vi "Main Tclk.vi"() -> ()   [LabVIEW 2018] (continued)
                        n6385 = invoke class="_EMApi" method="Execute"(reference=w1050, "lpszCommand"="CMD_FIB_TC_MH_REQ_START") -> ()  [unwired: 2 in, 4 out]
                      }
                      frame #2 {
                        n6386 = Wait (ms)(milliseconds to wait=u32 30000) -> ()  [unwired: 1 out]
                        n6387 = local write "Status message"("FIB reheat in progress..." ("Status message")) -> ()
                      }
                      frame #3 {
                        n6388 = while {
                          stop <- w1058 stop-if-true
                          n6389 = local read "Api"() -> (w1055:refnum<k7>)
                          n6390 = call "SmartSEM Remote API FIB gun state.vi"("ActiveX Container"=w1055) -> ("FIB Gun State"=w1057:string, "reference out"=w1053:refnum<k7>)  [unwired: 8 in, 1 out]
                          n6391 = Wait Until Next ms Multiple(millisecond multiple=u32 100) -> ()  [unwired: 1 out]
                          n6392 = case shown="\"FIB Emissin Failed\"" w1057 {
                            tunnel: [FALSE ("x") TRUE ("x") w1075] -> w1056
                            tunnel: w1053 -> [_ _ w1074]
                            frame "", Default {
                            }
                            frame "FIB Emissin Failed" {
                              n6393 = Get Date/Time In Seconds() -> (seconds since 1Jan1904=w1064:timestamp)
                              n6394 = Get Date/Time String(seconds (now)=w1064) -> (date string=w1065:string, time string=w1066:string)  [unwired: 2 in]
                              n6395 = Concatenate Strings(w1065, " " ("string"), w1066) -> (w1063:string)
                              n6396 = local read "Reheat Output"() -> (w1068:T21)
                              n6397 = Bundle By Name(cluster=w1068, "Reheat finish time"=w1063, "Reheat Success"=FALSE) -> (w1069:T21)
                              n6398 = local write "Reheat Output"(w1069) -> ()
                            }
                            frame "Regulating" {
                              n6399 = call "SmartSEM Remote API get string.vi"("lpszParam"="DP_FIB_PURGE_STATE", "ActiveX Container"=w1074) -> ("data"=w1072:string, "reference out"=w1071:refnum<k7>)  [unwired: 7 in, 1 out]
                              n6400 = case shown="\"Idle\"" w1072 {
                                tunnel: w1071 -> [_ w1078]
                                tunnel: [FALSE ("x") w1077] -> w1075
                                frame "", Default {
                                }
                                frame "Idle" {
                                n6401 = stacked-sequence {
                                tunnel: w1078 -> [w1081 _ w1086 _]
                                tunnel: [_ _ _ TRUE ("x")] -> w1077
                                frame #0 {
                                n6402 = local read "FIB HW Config"() -> (w1080:T23)
                                n6403 = Unbundle By Name(w1080) -> ("Beam blank"=w1079:tag)
                                n6404 = call "FIB beam blank.vi"("ActiveX Container"=w1081, "Beam blanked"=TRUE, "lines"=w1079) -> ()  [unwired: 2 in, 1 out]
                                }
                                frame #1 {
                                n6405 = Wait (ms)(milliseconds to wait=u32 60000) -> ()  [unwired: 1 out]
                                n6406 = local write "Status message"("Stablizing for 1 min ..." ("Status message")) -> ()
                                }
                                frame #2 {
                                n6407 = call "SmartSEM Remote API FIB VI slope.vi"("ActiveX Container"=w1086) -> ("V/I slope"=w1087:sgl)  [unwired: 8 in, 2 out]
                                n6408 = local write "Status message"("Measuring FIB V/I slope ..." ("Status message")) -> ()
                                n6409 = local write "FIB V/I slope"(w1087) -> ()
                                }
                                frame #3 {
                                }
                                }
                                }
                              }
                            }
                          }
                          n6410 = local read "Stop Reheat"() -> (w1054:bool)
                          n6411 = local read "Stop"() -> (w1060:bool)
                          n6412 = Compound Arithmetic op=OR(w1056, w1060, w1054) -> (w1058:bool)
                        }
                      }
                      frame #4 {
                        n6413 = while {
                          stop <- w1095 stop-if-true
                          n6414 = local read "Api"() -> (w1091:refnum<k7>)
                          n6415 = call "SmartSEM Remote API FIB gun state.vi"("ActiveX Container"=w1091) -> ("FIB Gun State"=w1094:string, "reference out"=w1089:refnum<k7>)  [unwired: 8 in, 1 out]
                          n6416 = Wait Until Next ms Multiple(millisecond multiple=u32 100) -> ()  [unwired: 1 out]
                          n6417 = case shown="\"Regulating\"" w1094 {
                            tunnel: [FALSE ("x") TRUE ("x") TRUE ("x") w1117] -> w1093
                            tunnel: w1089 -> [_ _ _ w1118]
                            frame "", Default {
                            }
                            frame "FIB Emissin Failed" {
                              n6418 = Get Date/Time In Seconds() -> (seconds since 1Jan1904=w1101:timestamp)
                              n6419 = Get Date/Time String(seconds (now)=w1101) -> (date string=w1102:string, time string=w1103:string)  [unwired: 2 in]
                              n6420 = Concatenate Strings(w1102, " " ("string"), w1103) -> (w1100:string)
                              n6421 = local read "Reheat Output"() -> (w1105:T21)
                              n6422 = Bundle By Name(cluster=w1105, "Reheat finish time"=w1100, "Reheat Success"=FALSE) -> (w1106:T21)
                              n6423 = local write "Reheat Output"(w1106) -> ()
                            }
                            frame "Standby" {
                              n6424 = Get Date/Time In Seconds() -> (seconds since 1Jan1904=w1110:timestamp)
                              n6425 = Get Date/Time String(seconds (now)=w1110) -> (date string=w1111:string, time string=w1112:string)  [unwired: 2 in]
                              n6426 = Concatenate Strings(w1111, " " ("string"), w1112) -> (w1109:string)
                              n6427 = local read "Reheat Output"() -> (w1114:T21)
                              n6428 = Bundle By Name(cluster=w1114, "Reheat finish time"=w1109, "Reheat Success"=FALSE) -> (w1115:T21)
                              n6429 = local write "Reheat Output"(w1115) -> ()
                            }
                            frame "Regulating" {
                              n6430 = stacked-sequence {
                                tunnel: w1118 -> [w1121 w1128]
                                tunnel: [_ w1129] -> w1117
                                frame #0 {
                                n6431 = Wait (ms)(milliseconds to wait=u32 2000) -> ()  [unwired: 1 out]
                                n6432 = call "SmartSEM Remote API set float.vi"("vValue"=sgl 1.0, "lpszParam"="DP_FIB_BLANKED", "ActiveX Container"=w1121) -> ("error out"=w1119:errorcluster, "reference out"=w1120:refnum<k7>)  [unwired: 7 in]
                                n6433 = call "SmartSEM Remote API get FIB HV data.vi"("error in"=w1119, "ActiveX Container"=w1120) -> ("Capella HV Data Output"=w1124:T17)  [unwired: 6 in, 3 out]
                                n6434 = local write "Capella HV Data Output"(w1124) -> ()
                                }
                                frame #1 {
                                n6435 = call "SmartSEM Remote API get string.vi"("lpszParam"="DP_FIB_PURGE_STATE", "ActiveX Container"=w1128) -> ("data"=w1126:string)  [unwired: 7 in, 2 out]
                                n6436 = case shown="\"Idle\"" w1126 {
                                tunnel: w1128 -> [_ w1132]
                                tunnel: [FALSE ("x") w1131] -> w1129
                                frame "", Default {
                                }
                                frame "Idle" {
                                n6437 = stacked-sequence {
                                tunnel: w1132 -> [_ w1143 _]
                                tunnel: [_ _ TRUE ("x")] -> w1131
                                frame #0 {
                                w1134 = TRUE ("Reheat Success")
                                n6438 = Get Date/Time In Seconds() -> (seconds since 1Jan1904=w1136:timestamp)
                                n6439 = local read "FIB V/I slope"() -> (w1133:sgl)
                                n6440 = Get Date/Time String(seconds (now)=w1136) -> (date string=w1137:string, time string=w1138:string)  [unwired: 2 in]
                                n6441 = Concatenate Strings(w1137, " " ("string"), w1138) -> (w1135:string)
                                n6442 = local read "Reheat Output"() -> (w1140:T21)
                                n6443 = Bundle By Name(cluster=w1140, "Reheat finish time"=w1135, "Reheat Success"=w1134, "V/I Slope"=w1133) -> (w1141:T21)
                                n6444 = local write "Start FIB HV DataLog"(w1134) -> ()
                                n6445 = local write "Reheat Output"(w1141) -> ()
                                }
                                frame #1 {
                                n6446 = call "SmartSEM Remote API FIB Gun Valve.vi"("FIB Gun Valve"=enum16{"Close", "Open"}."Open", "ActiveX Container"=w1143) -> ()  [unwired: 8 in, 2 out]
                                }
                                frame #2 {
                                n6447 = local read "Reheat Output"() -> (w1148:T21)
                                n6448 = local read "Capella HV Data Output"() -> (w1146:T17)
                                n6449 = Unbundle By Name(w1146) -> ("Emission Actual (uA)"=w1145:sgl, "Suppressor (V)"=w1144:sgl)
                                n6450 = Bundle By Name(cluster=w1148, "Initial emission (uA)"=w1145, "Initial suppressor (V)"=w1144) -> (w1147:T21)
                                n6451 = local write "Reheat Output"(w1147) -> ()
                                }
                                }
                                }
                                }
                                }
                              }
                            }
                          }
                          n6452 = local write "Status message"("Finishing FIB reheat ..." ("Status message")) -> ()
                          n6453 = local read "Stop Reheat"() -> (w1090:bool)
                          n6454 = local read "Stop"() -> (w1097:bool)
                          n6455 = Compound Arithmetic op=OR(w1093, w1097, w1090) -> (w1095:bool)
                        }
                      }
                      frame #5 {
                        n6456 = local read "Stop Reheat"() -> (w1150:bool)
                        n6457 = case shown="False" w1150 {
                          frame False {
                            n6458 = local read "Api"() -> (w1152:refnum<k7>)
                            n6459 = call "SmartSEM Remote API FIB HV offset removal.vi"("Max offset threshold (V)"=sgl 80.0, "ActiveX Container"=w1152) -> ("FIB HV matched"=w1151:bool)  [unwired: 8 in, 1 out]
                            n6460 = local write "FIB HV target matched"(w1151) -> ()
                          }
                          frame True {
                          }
                        }
                      }
                      frame #6 {
                        n6461 = local read "Stop Reheat"() -> (w1154:bool)
                        n6462 = case shown="False" w1154 {
                          tunnel: w1155 -> [w1157 w1162]
                          frame False {
                            n6463 = local read "Reheat Output"() -> (w1160:T21)
                            n6464 = local read "FIB Reheat Log Files"() -> (w1159:path)
                            n6465 = local read "Reheat time"() -> (w1158:timestamp)
                            n6466 = local read "Capella HV Data Output"() -> (w1156:T17)
                            n6467 = local write "Status message"("FIB reheat completed" ("Status message")) -> ()
                            n6468 = call "Write FIB reheat log.vi"("Capella HV Data Output"=w1156, "Reheat Output"=w1160, "Reheat time"=w1158, "Machine Type"=w1157, "Log file path"=w1159) -> ()  [unwired: 7 in]
                          }
                          frame True {
                            n6469 = local read "Reheat Output"() -> (w1165:T21)
                            n6470 = local read "FIB Reheat Log Files"() -> (w1164:path)
                            n6471 = local read "Reheat time"() -> (w1163:timestamp)
                            n6472 = local write "Status message"("FIB reheat stopped" ("Status message")) -> ()
                            n6473 = call "Write FIB reheat log.vi"("Reheat Output"=w1165, "Reheat time"=w1163, "Machine Type"=w1162, "Log file path"=w1164) -> ()  [unwired: 8 in]
                          }
                        }
                      }
                    }
                  }
                }
              }
              frame #2 {
                w1167 = u8 0 ("FIB emission below limit counts")
                w1170 = FALSE ("Start Reheat")
                n6474 = local write "Start Reheat"(w1170) -> ()
                n6475 = local write "Stop Reheat"(w1170) -> ()
                n6476 = local write "Turn FIB Gun on"(w1170) -> ()
                n6477 = property on="Request to stop reheat" class="Bool (strict)"("DisabledEnum"=T44."Disabled and Grayed Out" ("Disabled")) -> ()  [unwired: 2 in, 2 out]
                n6478 = local write "FIB emission limit warning armed"(TRUE ("FIB emission limit warning armed")) -> ()
                n6479 = local write "FIB emission below limit counts"(w1167) -> ()
                n6480 = local write "FIB suppressor below limit counts"(w1167) -> ()
                "Reheat completed" <- TRUE ("Reheat completed")
              }
            }
          }
        }
        n6481 = local read "Stop"() -> (w889:bool)
      }
      n6482 = while {
        stop <- w5736 stop-if-true
        n6483 = stacked-sequence {
          tunnel: [_ w5783] -> w5736
          frame #0 {
            n6484 = local read "Spot"() -> (w5739:bool)
            n6485 = shared-variable "My Computer\\Zeiss Library.lvlib\\Spot"(w5739) -> ()  [unwired: 1 in, 1 out]
            n6486 = local read "Machine Type"() -> (w5738:u8)
            n6487 = case shown="True" w5739 {
              tunnel: w5738 -> [_ w5741]
              frame False {
                n6488 = shared-variable ".\\Zeiss Library.lvlib\\FIB spot mode"(FALSE ("FIB spot mode")) -> ()  [unwired: 1 in, 1 out]
              }
              frame True {
                n6489 = stacked-sequence {
                  tunnel: w5741 -> [_ _ _ _ w5764 _ _]
                  frame #0 {
                    w5743 = 5.0 ("Cursor.Cursor Position:Cursor X")
                    w5742 = FALSE ("Unfreeze")
                    w5744 = TRUE ("Realtime Imaging stop")
                    n6490 = shared-variable "My Computer\\Zeiss Library.lvlib\\Realtime Imaging stop"(w5744) -> ()  [unwired: 1 in, 1 out]
                    n6491 = shared-variable ".\\Zeiss Library.lvlib\\FIB spot mode"(w5744) -> ()  [unwired: 1 in, 1 out]
                    n6492 = property on="FIB Imaging" class="Bool (strict)"("DisabledEnum"=T44."Disabled and Grayed Out" ("Disabled")) -> ()  [unwired: 2 in, 2 out]
                    n6493 = property on="FIB Image" class="IntGraph (strict)"() -> ("Width"=w5746:u32, "Height"=w5747:u32)  [unwired: 2 in, 2 out]
                    n6494 = expression code="x/2"(w5746) -> ()  [unwired: 1 out]
                    n6495 = expression code="x/2"(w5747) -> ()  [unwired: 1 out]
                    n6496 = local write "FIB Imaging"(w5742) -> ()
                    n6497 = local write "Unfreeze"(w5742) -> ()
                    n6498 = property on="FIB Image" class="IntGraph (strict)"("Cursor.Cursor X"=w5743, "Cursor.Cursor Y"=w5743) -> ()  [unwired: 2 in, 2 out]
                  }
                  frame #1 {
                    w5748 = -0.99 ("Spot X")
                    n6499 = Wait (ms)(milliseconds to wait=u32 500) -> ()  [unwired: 1 out]
                    n6500 = shared-variable ".\\Zeiss Library.lvlib\\Spot X"(w5748) -> ()  [unwired: 1 in, 1 out]
                    n6501 = shared-variable "My Computer\\Zeiss Library.lvlib\\Spot Z"(w5748) -> ()  [unwired: 1 in, 1 out]
                  }
                  frame #2 {
                    n6502 = local read "FIB HW Config"() -> (w5752:T23)
                    n6503 = local read "Api"() -> (w5750:refnum<k7>)
                    n6504 = local read "FIB Scan Parameters"() -> (w5751:T32)
                    n6505 = local read "FIB Options"() -> (w5756:T33)
                    n6506 = Unbundle By Name(w5756) -> ("Flip x"=w5755:bool, "Flip z"=w5754:bool)
                    n6507 = Bundle("Flip x"=w5755, "Flip z"=w5754) -> (w5753:cluster{"Flip x":bool, "Flip z":bool})  [unwired: 1 in]
                    n6508 = call "FIB spot PXIe-6124.vi"("FIB Scan Parameters"=w5751, "ActiveX Container"=w5750, "Options"=w5753, "HW Config"=w5752) -> ("error out"=w5758:errorcluster)  [unwired: 7 in]
                    n6509 = Unbundle By Name(w5758) -> ("status"=w5757:bool)
                    n6510 = case shown="True" w5757 {
                      frame False {
                      }
                      frame True {
                        n6511 = local write "Spot"(FALSE ("Spot")) -> ()
                      }
                    }
                  }
                  frame #3 {
                    n6512 = disable-structure shown="Disabled" {
                      frame Disabled {
                        w5763 = TRUE ("Unfreeze")
                        n6513 = local write "FIB Imaging"(w5763) -> ()
                        n6514 = local write "Unfreeze"(w5763) -> ()
                      }
                      frame Enabled {
                      }
                    }
                    n6515 = shared-variable ".\\Zeiss Library.lvlib\\FIB spot mode"(FALSE ("Realtime Imaging stop")) -> ()  [unwired: 1 in, 1 out]
                    n6516 = property on="FIB Imaging" class="Bool (strict)"("DisabledEnum"=T44."Enabled" ("Disabled")) -> ()  [unwired: 2 in, 2 out]
                    n6517 = property on="Spot" class="Bool (strict)"("DisabledEnum"=T44."Disabled and Grayed Out" ("Disabled")) -> ()  [unwired: 2 in, 2 out]
                  }
                  frame #4 {
                    n6518 = case shown="2" w5764 {
                      frame 0, Default {
                      }
                      frame 1 {
                        w5766 = TRUE ("Initialization")
                        n6519 = local read "COM port"() -> (w5765:refnum<visa-resource-name>)
                        n6520 = call "FIB mode.vi"("Initialization"=w5766, "FIB mode"=T10."SEM", "COM port in"=w5765) -> ("COM port out"=w5771:refnum<visa-resource-name>)  [unwired: 7 in, 1 out]
                        n6521 = call "Remcon32 command.vi"("SEM command"="edx 0", "COM port in"=w5771) -> ("COM port out"=w5770:refnum<visa-resource-name>)  [unwired: 6 in, 3 out]
                        n6522 = call "Remcon32 command.vi"("Close session"=w5766, "SEM command"="frez", "COM port in"=w5770) -> ()  [unwired: 5 in, 4 out]
                      }
                      frame 2 {
                        n6523 = local read "Api"() -> (w5772:refnum<k7>)
                        n6524 = call "SmartSEM Remote API set float.vi"("vValue"=sgl 2.0, "lpszParam"="DP_FIB_BLANKER_MODE" ("lpszCommand"), "ActiveX Container"=w5772) -> ("error out"=w5780:errorcluster, "reference out"=w5779:refnum<k7>)  [unwired: 7 in]
                        n6525 = call "SmartSEM Remote API FIB mode.vi"("error in"=w5780, "FIB mode"=T50."SEM", "ActiveX Container"=w5779) -> ("error out"=w5776:errorcluster, "reference out"=w5775:refnum<k7>)  [unwired: 7 in]
                        n6526 = invoke class="_EMApi" method="Execute"(reference=w5775, error in=w5776, "lpszCommand"="CMD_FREEZE_ALL") -> ()  [unwired: 1 in, 4 out]
                      }
                    }
                  }
                  frame #5 {
                    n6527 = Wait (ms)(milliseconds to wait=u32 4000) -> ()  [unwired: 1 out]
                  }
                  frame #6 {
                    n6528 = property on="Spot" class="Bool (strict)"("DisabledEnum"=T44."Enabled" ("Disabled")) -> ()  [unwired: 2 in, 2 out]
                  }
                }
              }
            }
          }
          frame #1 {
            n6529 = local read "Stop"() -> (w5783:bool)
          }
        }
        n6530 = Wait Until Next ms Multiple(millisecond multiple=u32 100) -> ()  [unwired: 1 out]
      }
      n6531 = while {
        stop <- w2544 stop-if-true
        n6532 = case shown="True" "Scan xn" {
          tunnel: [w2546 w2547] -> w2544
          frame False {
            n6533 = local read "Stop"() -> (w2546:bool)
          }
          frame True {
            n6534 = while {
              tunnel: [w2550] -> w2547
              stop <- w2552 stop-if-true
              n6535 = stacked-sequence {
                seq-local: [_ w2572 _ _ _] -> [_ _ w2581 _ _]
                seq-local: [_ _ w2590 _ _] -> [_ _ _ w2596 _]
                seq-local: [_ _ w2589 _ _] -> [_ _ _ w2597 _]
                frame #0 {
                  w2557 = u32 3600 ("upper limit")
                  w2561 = u32 600 ("upper limit")
                  w2553 = u32 0 ("lower limit")
                  n6536 = local read "SEM-FIB Delay (s)"() -> (w2556:u32)
                  n6537 = In Range and Coerce(upper limit=u32 36000, x=w2556, lower limit=w2557) -> (In Range?=w2555:bool)  [unwired: 1 out]
                  n6538 = In Range and Coerce(upper limit=w2557, x=w2556, lower limit=w2561) -> (In Range?=w2559:bool)  [unwired: 1 out]
                  n6539 = In Range and Coerce(upper limit=w2561, x=w2556, lower limit=w2553) -> (In Range?=w2560:bool)  [unwired: 1 out]
                  n6540 = Build Array(w2555, w2559, w2560) -> (w2563:bool[])
                  n6541 = local read "Additional Info"() -> (w2565:cluster{"Restart flag":u8, "Stage move flag":u8})
                  n6542 = Boolean Array To Number(Boolean array=w2563) -> (number=w2562:u32)
                  n6543 = case shown="2" w2562 {
                    tunnel: [u32 100 ("lower limit") u32 10 ("lower limit") u32 2 ("lower limit") u32 0 ("lower limit")] -> w2554
                    frame 0, Default {
                    }
                    frame 1 {
                    }
                    frame 2 {
                    }
                    frame 4 {
                    }
                  }
                  n6544 = Bundle By Name(cluster=w2565, "Restart flag"=w2554, "Stage move flag"=w2553) -> (w2564:cluster{"Restart flag":u8, "Stage move flag":u8})
                  n6545 = local write "Additional Info"(w2564) -> ()
                }
                frame #1 {
                  n6546 = local read "Tiled scan inputs"() -> (w2573:T6)
                  n6547 = local read "SEM HW Config"() -> (w2574:T9)
                  n6548 = local read "Detector Information"() -> (w2575:T8)
                  n6549 = local read "SEM Scan Parameters"() -> (w2576:T26)
                  n6550 = local read "SEM Options"() -> (w2577:T27)
                  n6551 = local read "Focus Index Options"() -> (w2571:T28)
                  n6552 = local read "File Information"() -> (w2578:T31)
                  n6553 = local read "Milling para"() -> (w2579:T35)
                  n6554 = local read "Additional Info"() -> (w2570:cluster{"Restart flag":u8, "Stage move flag":u8})
                  n6555 = Bundle By Name(cluster=w2573, "HW Config"=w2574, "Det Info"=w2575, "SEM Scan Parameters"=w2576, "SEM Options"=w2577, "Focus Index Options"=w2571, "File Information"=w2578, "Milling para"=w2579, "Additional Info"=w2570) -> (w2572:T6)
                }
                frame #2 {
                  n6556 = local read "Api"() -> (w2580:refnum<k7>)
                  n6557 = local read "WatchDog Mode"() -> (w2582:u16)
                  n6558 = call "2D scan tiled.vi"("WatchDog Mode"=w2582, "Tiled scan inputs"=w2581, "ActiveX Container"=w2580) -> ("Image Focus Index Tiled"=w2589:T53, "Image Focus Index Array Tiled"=w2590:T54, "Single scan outputs"=w2593:T55, "8-bit over scale"=w2583:bool[])  [unwired: 3 in, 2 out]
                  n6559 = Unbundle By Name(w2593) -> ("SEM Parameters"=w2592:T13, "Image Focus Index"=w2591:T14)
                  n6560 = Index Array(array=w2583, index #1=0 ("index"), index #2=1 ("index")) -> (element #1=w2586:bool, element #2=w2587:bool)
                  n6561 = local write "SEM Parameters"(w2592) -> ()
                  n6562 = local write "Image Focus Index"(w2591) -> ()
                  n6563 = local write "Det A over scale"(w2586) -> ()
                  n6564 = local write "Det B over scale"(w2587) -> ()
                  n6565 = local write "Status message"("SEM scanning" ("Status message")) -> ()
                }
                frame #3 {
                  n6566 = local read "FI Detector"() -> (w2598:u16)
                  n6567 = case shown="0, Default" w2598 {
                    tunnel: w2597 -> [w2602 w2606 w2610 w2614]
                    tunnel: [w2601 w2603 w2609 w2613] -> w2595
                    tunnel: w2596 -> [w2599 w2605 w2608 w2612]
                    tunnel: [w2600 w2604 w2607 w2611] -> w2594
                    frame 0, Default {
                      n6568 = Unbundle By Name(w2602) -> ("A Img Focus Index"=w2601:sgl[][])
                      n6569 = Unbundle By Name(w2599) -> ("A Img Focus Index array"=w2600:sgl[][][][])
                    }
                    frame 1 {
                      n6570 = Unbundle By Name(w2606) -> ("B Img Focus Index"=w2603:sgl[][])
                      n6571 = Unbundle By Name(w2605) -> ("B Img Focus Index array"=w2604:sgl[][][][])
                    }
                    frame 2 {
                      n6572 = Unbundle By Name(w2610) -> ("C Img Focus Index"=w2609:sgl[][])
                      n6573 = Unbundle By Name(w2608) -> ("C Img Focus Index array"=w2607:sgl[][][][])
                    }
                    frame 3 {
                      n6574 = Unbundle By Name(w2614) -> ("D Img Focus Index"=w2613:sgl[][])
                      n6575 = Unbundle By Name(w2612) -> ("D Img Focus Index array"=w2611:sgl[][][][])
                    }
                  }
                  n6576 = local write "Focus Index array tiled"(w2594) -> ()
                  n6577 = local write "Focus Index tiled"(w2595) -> ()
                }
                frame #4 {
                  n6578 = local read "Scan xn"() -> (w2615:bool)
                  n6579 = case shown="False" w2615 {
                    tunnel: ["SEM scanning pause" ("Status message") "SEM scanning finished" ("Status message")] -> w2616
                    frame True {
                    }
                    frame False {
                    }
                  }
                  n6580 = local write "Status message"(w2616) -> ()
                  n6581 = Wait (ms)(milliseconds to wait=u32 1000) -> ()  [unwired: 1 out]
                }
              }
              n6582 = Wait Until Next ms Multiple(millisecond multiple=u32 100) -> ()  [unwired: 1 out]
              n6583 = local read "Scan xn"() -> (w2551:bool)
              n6584 = Not(x=w2551) -> (.not. x?=w2549:bool)
              n6585 = local read "Stop"() -> (w2550:bool)
              n6586 = Or(x=w2549, y=w2550) -> (x .or. y?=w2552:bool)
            }
          }
        }
        n6587 = Wait Until Next ms Multiple(millisecond multiple=u32 100) -> ()  [unwired: 1 out]
      }
      n6588 = while {
        stop <- w3128 stop-if-true
        w3135 = -1.0 ("lower limit")
        w3136 = 1.0 ("upper limit")
        n6589 = property on="FIB Image" class="IntGraph (strict)"() -> ("Cursor.Cursor X"=w3130:dbl, "Width"=w3129:u32, "Cursor.Cursor Y"=w3132:dbl, "Height"=w3131:u32)  [unwired: 2 in, 2 out]
        n6590 = local read "Stop"() -> (w3128:bool)
        n6591 = Wait Until Next ms Multiple(millisecond multiple=u32 100) -> ()  [unwired: 1 out]
        n6592 = Not(x=w3128) -> (.not. x?=w3126:bool)
        n6593 = expression code="x/2"(w3129) -> (w3134:u32)
        n6594 = expression code="x/2"(w3131) -> (w3133:u32)
        n6595 = Compound Arithmetic op=AND("Spot", w3126) -> (w3146:bool)
        n6596 = shared-variable "My Computer\\Zeiss Library.lvlib\\Milling Manual Pause"("Mill Manual Pause") -> (error out=w3125:errorcluster)  [unwired: 1 in]
        n6597 = shared-variable "My Computer\\Zeiss Library.lvlib\\Milling Stop"("Mill Stop", error in=w3125) -> (error out=w3124:errorcluster)
        n6598 = shared-variable ".\\Zeiss Library.lvlib\\FIB beam blank"("Beam blanked", error in=w3124) -> (error out=w3123:errorcluster)
        n6599 = property on="FIB Image" class="IntGraph (strict)"("Cursor.Visible"="Spot") -> ()  [unwired: 2 in, 2 out]
        n6600 = Subtract(x=w3130, y=w3134) -> (x-y=w3142:dbl)
        n6601 = Subtract(x=w3132, y=w3133) -> (x-y=w3141:dbl)
        n6602 = Divide(x=w3142, y=w3134) -> (x/y=w3140:dbl)
        n6603 = Divide(x=w3141, y=w3133) -> (x/y=w3137:dbl)
        n6604 = In Range and Coerce(upper limit=w3136, x=w3140, lower limit=w3135) -> (coerced(x)=w3139:dbl)  [unwired: 1 out]
        n6605 = In Range and Coerce(upper limit=w3136, x=w3137, lower limit=w3135) -> (coerced(x)=w3138:dbl)  [unwired: 1 out]
        n6606 = shared-variable ".\\Zeiss Library.lvlib\\Spot X"(w3139, error in=w3123) -> (error out=w3122:errorcluster)
        n6607 = shared-variable "My Computer\\Zeiss Library.lvlib\\Spot Z"(w3138, error in=w3122) -> (error out=w3121:errorcluster)
        n6608 = shared-variable ".\\Zeiss Library.lvlib\\FIB spot mode"(w3146, error in=w3121) -> ()  [unwired: 1 out]
      }
      n6609 = while {
        stop <- w5717 stop-if-true
        n6610 = case shown="True" "Mill" {
          frame False {
            n6611 = property on="FIB Imaging" class="Bool (strict)"("DisabledEnum"=T44."Enabled" ("Disabled")) -> ()  [unwired: 2 in, 2 out]
          }
          frame True {
            n6612 = stacked-sequence {
              frame #0 {
                w5720 = FALSE ("Freeze")
                n6613 = local write "Unfreeze"(w5720) -> ()
                n6614 = local write "Mill Manual Pause"(w5720) -> ()
                n6615 = local write "Mill Stop"(w5720) -> ()
              }
              frame #1 {
                n6616 = Wait (ms)(milliseconds to wait=u32 500) -> ()  [unwired: 1 out]
              }
              frame #2 {
                n6617 = local read "WatchDog Mode"() -> (w5723:u16)
                n6618 = local read "Api"() -> (w5722:refnum<k7>)
                n6619 = local read "FIB Scan Parameters"() -> (w5728:T32)
                n6620 = local read "FIB HW Config"() -> (w5729:T23)
                n6621 = local read "FIB Options"() -> (w5733:T33)
                n6622 = local read "Machine Type"() -> (w5726:u8)
                n6623 = Unbundle By Name(w5733) -> ("Flip x"=w5732:bool, "Flip z"=w5731:bool)
                n6624 = local read "Damping"() -> (w5724:bool)
                n6625 = local read "COM port"() -> (w5727:refnum<visa-resource-name>)
                n6626 = Bundle("Flip x"=w5732, "Flip z"=w5731) -> (w5730:cluster{"Flip x":bool, "Flip z":bool})  [unwired: 1 in]
                n6627 = call "FIB trapezoidal mill PXIe-6124.vi"("ActiveX Container"=w5722, "COM port"=w5727, "WatchDog Mode"=w5723, "FIB Scan Parameters"=w5728, "FIB HW Config"=w5729, "Options"=w5730, "Milling para"="Milling para", "Machine Type"=w5726, "Damping"=w5724) -> ()  [unwired: 3 in, 4 out]
              }
              frame #3 {
                n6628 = shared-variable "My Computer\\Zeiss Library.lvlib\\Milling Line Paused"(TRUE ("Rect Milling Line Paused")) -> ()  [unwired: 1 in, 1 out]
                n6629 = local write "Mill"(FALSE ("Mill")) -> ()
              }
            }
          }
        }
        n6630 = Wait Until Next ms Multiple(millisecond multiple=u32 100) -> ()  [unwired: 1 out]
        n6631 = local read "Stop"() -> (w5717:bool)
      }
      n6632 = while {
        stop <- w1921 stop-if-true
        n6633 = Wait Until Next ms Multiple(millisecond multiple=u32 100) -> ()  [unwired: 1 out]
        n6634 = case shown="True" "Enable logging" {
          frame False {
          }
          frame True {
            n6635 = stacked-sequence {
              frame #0 {
                n6636 = Get Date/Time In Seconds() -> (seconds since 1Jan1904=w1927:timestamp)
                n6637 = Reciprocal(x="Sample rate (Hz)") -> (1/x=w1924:dbl)
                n6638 = To Double Precision Float(number=w1927) -> (double precision float=w1926:dbl)
                n6639 = property on="Measurements" class="WFChart (strict)"("History Data"=dbl[][] [], "XScale.Offset"=w1926, "XScale.Multiplier"=w1924) -> ()  [unwired: 2 in, 2 out]
              }
              frame #1 {
                w1943 = 10123 items=["Finite Samples"=10178, "Continuous Samples"=10123, "Hardware Timed Single Point"=12522] ("sample mode")
                n6640 = local read "Sample rate (Hz)"() -> (w1933:dbl)
                n6641 = local read "Active logging channels"() -> (w1932:string)
                n6642 = call-poly <vilib>:"DAQmx Create Virtual Channel.vi"("physical channels"=w1932) -> ("task out"=w1942:refnum<k21>, "error out"=w1941:errorcluster)  [unwired: 13 in]
                n6643 = call-poly <vilib>:"DAQmx Timing.vi"("task/channels in"=w1942, "sample mode"=w1943, "rate"=w1933, "error in"=w1941) -> ("task out"=w1930:refnum<k21>, "error out"=w1939:errorcluster)  [unwired: 10 in]
                n6644 = local read "Machine Type"() -> (w1929:u8)
                n6645 = call <vilib>:"DAQmx Configure Input Buffer.vi"("task/channels in"=w1930, "buffer size (in samples per channel)"=u32 1000000, "error in"=w1939) -> ("task out"=w1940:refnum<k21>, "error out"=w1938:errorcluster)  [unwired: 11 in]
                n6646 = call <vilib>:"DAQmx Start Task.vi"("task/channels in"=w1940, "error in"=w1938) -> ("task out"=w1935:refnum<k21>, "error out"=w1934:errorcluster)  [unwired: 12 in]
                n6647 = while {
                  tunnel: w1934 -> [w1982]
                  tunnel: w1935 -> [w1981]
                  tunnel: [w1980] -> w1936
                  tunnel: [w1979] -> w1937
                  tunnel: w1929 -> [w1957]
                  tunnel: "Samples size" -> [w1955]
                  shift-right: [w1949] -> _
                  shift-left: _ -> [w1947]
                  stop <- w1975 stop-if-true
                  # "Last 1.5 seconds of Specimen Current"
                  # "10 Hz"
                  n6648 = local read "Faraday Cup before mill"() -> (w1964:sgl)
                  n6649 = call-poly <vilib>:"DAQmx Read.vi"("task/channels in"=w1981, "number of samples per channel"=w1955, "error in"=w1982) -> ("task out"=w1980:refnum<k21>, "data"=w1973:dbl[][], "error out"=w1979:errorcluster)  [unwired: 10 in]
                  n6650 = To Single Precision Float(number=w1973) -> (single precision float=w1972:sgl[][])
                  n6651 = expression code="x*10"(w1972) -> (w1956:sgl[][])
                  n6652 = case shown="2" w1957 {
                    tunnel: w1956 -> [w1983 w1986]
                    tunnel: w1955 -> [_ w1985]
                    tunnel: [w1983 w1984] -> w1950
                    frame 0, Default {
                    }
                    frame 2 {
                      n6653 = local read "Api"() -> (w1987:refnum<k7>)
                      n6654 = call "SmartSEM Remote API FIB Faraday cup.vi"("ActiveX Container"=w1987) -> ("FIB Faraday Cup (nA)"=w1988:sgl)  [unwired: 8 in, 2 out]
                      n6655 = Initialize Array(w1988, w1985) -> (w1989:sgl[])
                      n6656 = Replace Array Subset(array=w1986, new element=w1989) -> (w1984:sgl[][])  [unwired: 2 in]
                    }
                  }
                  "Measurements" <- w1950
                  n6657 = To Single Precision Float(number=w1950) -> (single precision float=w1954:sgl[][])
                  n6658 = call "2D Array Decimate.vi"("x decimating factor"=w1955, "Input 2D Array"=w1950) -> ("output array"=w1971:dbl[][])  [unwired: 7 in, 2 out]
                  n6659 = To Single Precision Float(number=w1971) -> (single precision float=w1970:sgl[][])
                  n6660 = Index Array(array=w1954, index (row)=1 ("index")) -> (element=w1948:sgl[])  [unwired: 1 in]
                  n6661 = Index Array(array=w1970, index (col)=0 ("disabled index (col)")) -> (element=w1966:sgl[])  [unwired: 1 in]
                  n6662 = Build Array (concatenate)(w1947, w1948) -> (w1945:sgl[])
                  n6663 = Array Size(array=w1945) -> (size(s)=w1953:i32)
                  n6664 = Subtract(x=w1953, y=1500) -> (x-y=w1946:i32)
                  n6665 = Index Array(array=w1966, index #1=3 ("index"), index #2=2 ("index"), index #3=1 ("index"), index #4=0 ("index")) -> (element #1=→"BD2 RT":sgl, element #2=w1963:sgl, element #3=→"Specimen RT":sgl, element #4=→"Faraday Cup RT":sgl)
                  "BD1 RT" <- w1963
                  n6666 = Array Subset(array=w1945, index=w1946) -> (w1949:sgl[])  [unwired: 1 in]
                  n6667 = local read "Enable logging"() -> (w1978:bool)
                  n6668 = shared-variable ".\\Zeiss Library.lvlib\\Log For Shutter"(w1949) -> ()  [unwired: 1 in, 1 out]
                  n6669 = Subtract(x=w1964, y=w1963) -> (x-y=w1967:sgl)
                  n6670 = local read "Stop"() -> (w1976:bool)
                  n6671 = Build Array (concatenate)(w1966, w1967) -> (w1965:sgl[])
                  n6672 = shared-variable ".\\Zeiss Library.lvlib\\Logs"(w1965) -> ()  [unwired: 1 in, 1 out]
                  n6673 = Not(x=w1978) -> (.not. x?=w1977:bool)
                  n6674 = Or(x=w1977, y=w1976) -> (x .or. y?=w1975:bool)
                }
                n6675 = call <vilib>:"DAQmx Clear Task.vi"("task in"=w1936, "error in"=w1937) -> ("error out"=w1931:errorcluster)  [unwired: 13 in]
                n6676 = call <vilib>:"General Error Handler.vi"("error in (no error)"=w1931) -> ()  [unwired: 10 in, 5 out]
              }
            }
          }
        }
        n6677 = local read "Stop"() -> (w1921:bool)
      }
      n6678 = while {
        shift-right: [w1991] -> _
        shift-left: _ -> [w1990]
        stop <- w1993 stop-if-true
        n6679 = stacked-sequence {
          tunnel: [_ _ _ _ _ _ _ _ _ _ _ _ _ _ _ _ _ w2337 _ _ _ _ _ _ _ _ _] -> w1991
          tunnel: w1990 -> [_ _ _ _ _ _ _ _ _ _ _ _ _ _ _ _ _ w2338 w2355 w2373 _ _ _ _ _ _ _]
          frame #0 {
            n6680 = local read "FIB slice #"() -> (w1998:u32)
            n6681 = Not Equal To 0?(x="Images per Auto Optimization") -> (x != 0?=w1995:bool)
            n6682 = Not Equal To 0?(x=w1998) -> (x != 0?=w1999:bool)
            n6683 = Compound Arithmetic op=AND("Auto Optimzation", w1995, w1999) -> (w1994:bool)
            n6684 = case shown="True" w1994 {
              frame False {
              }
              frame True {
                n6685 = local read "WD array tiled"() -> (w2005:sgl[][][])
                n6686 = local read "StigX array tiled"() -> (w2003:sgl[][][])
                n6687 = local read "StigY array tiled"() -> (w2002:sgl[][][])
                n6688 = local read "AF Steps"() -> (w2021:u8)
                n6689 = local read "FIB slice #"() -> (w2015:u32)
                n6690 = local read "Images per Auto Optimization"() -> (w2019:u16)
                n6691 = Empty Array?(array=w2005) -> (empty?=w2004:bool)
                n6692 = Empty Array?(array=w2003) -> (empty?=w2001:bool)
                n6693 = Empty Array?(array=w2002) -> (empty?=w2000:bool)
                n6694 = local read "AF Success tiled"() -> (w2007:bool[][])
                n6695 = Increment(x=w2021) -> (x+1=w2020:u8)
                n6696 = And(x=w2001, y=w2000) -> (x .and. y?=w2008:bool)
                n6697 = local read "Auto Stig"() -> (w2012:bool)
                n6698 = local read "Auto Align"() -> (w2010:bool)
                n6699 = Quotient & Remainder(x=w2015, y=w2019) -> (x-y*floor(x/y)=w2022:u32)  [unwired: 1 out]
                n6700 = And Array Elements(Boolean array=w2007) -> (logical AND=w2006:bool)
                n6701 = Equal?(x=w2020, y=w2022) -> (x = y?=w2014:bool)
                n6702 = Not Equal To 0?(x=w2015) -> (x != 0?=w2016:bool)
                n6703 = Equal To 0?(x=w2022) -> (x = 0?=w2017:bool)
                n6704 = Not(x=w2012) -> (.not. x?=w2011:bool)
                n6705 = Not(x=w2010) -> (.not. x?=w2009:bool)
                n6706 = Compound Arithmetic op=AND(w2004, w2006, w2014, w2009) -> (w2013:bool)
                n6707 = Compound Arithmetic op=AND(w2016, w2017, w2008, w2011, w2009) -> (w2018:bool)
                n6708 = case shown="True" w2013 {
                  frame False {
                  }
                  frame True {
                    n6709 = local write "Auto Stig"(TRUE ("Auto Focus")) -> ()
                  }
                }
                n6710 = case shown="True" w2018 {
                  frame False {
                  }
                  frame True {
                    n6711 = local write "Auto Focus"(TRUE ("Auto Focus")) -> ()
                  }
                }
              }
            }
          }
          frame #1 {
            n6712 = local read "Email Alert Recipients"() -> (w2028:string[])
            n6713 = local read "Mail server"() -> (w2029:string)
            n6714 = local read "Hardware Configuration"() -> (w2031:T25)
            n6715 = local read "Email Log Files"() -> (w2025:path)
            n6716 = Unbundle By Name(w2031) -> ("Machine ID"=w2030:string)
            n6717 = call "Email alert.vi"("Email log file path"=w2025, "Send email"="E-mail test", "Machine ID"=w2030, "Mail server"=w2029, "Alarm message"="E-mail test", "Recipents"=w2028) -> ()  [unwired: 6 in]
            n6718 = case shown="True" "E-mail test" {
              frame False {
              }
              frame True {
                n6719 = stacked-sequence {
                  frame #0 {
                    n6720 = Wait (ms)(milliseconds to wait=u32 200) -> ()  [unwired: 1 out]
                  }
                  frame #1 {
                    n6721 = local write "E-mail test"(FALSE ("E-mail test")) -> ()
                  }
                }
              }
            }
          }
          frame #2 {
            n6722 = local read "Machine Type"() -> (w2042:u8)
            n6723 = case shown="2" w2042 {
              tunnel: [w2052 w2054 w2056] -> w2043
              frame 0, Default {
                n6724 = local read "HV Data Output"() -> (w2053:T18)
                n6725 = Unbundle By Name(w2053) -> ("Emission (uA)"=w2052:sgl)
              }
              frame 1 {
                n6726 = local read "FIB Parameters"() -> (w2055:T19)
                n6727 = Unbundle By Name(w2055) -> ("FIB emission (uA)"=w2054:sgl)
              }
              frame 2 {
                n6728 = local read "Capella HV Data Output"() -> (w2057:T17)
                n6729 = Unbundle By Name(w2057) -> ("Emission Actual (uA)"=w2056:sgl)
              }
            }
            n6730 = local read "Alert Settings"() -> (w2040:T36)
            n6731 = local read "FIB"() -> (w2034:bool)
            n6732 = local read "FIB emission limit warning active"() -> (w2045:bool)
            n6733 = local read "FIB emission limit warning armed"() -> (w2046:bool)
            n6734 = Unbundle By Name(w2040) -> ("FIB emission warning"=w2039:bool)
            n6735 = Format Into String(format string="%4.2f", w2043) -> (resulting string=w2044:string)  [unwired: 2 in, 1 out]
            n6736 = Concatenate Strings("FIB emission reached ", w2044, "uA" ("resulting string")) -> (w2041:string)
            n6737 = case shown="True" w2045 {
              frame False {
              }
              frame True {
                n6738 = stacked-sequence {
                  frame #0 {
                    n6739 = Wait (ms)(milliseconds to wait=u32 500) -> ()  [unwired: 1 out]
                  }
                  frame #1 {
                    "FIB emission limit warning armed" <- FALSE ("3D image paused active bypass")
                  }
                }
              }
            }
            n6740 = local read "Email Alert Recipients"() -> (w2047:string[])
            n6741 = local read "Mail server"() -> (w2048:string)
            n6742 = local read "Hardware Configuration"() -> (w2051:T25)
            n6743 = local read "Email Log Files"() -> (w2038:path)
            n6744 = Compound Arithmetic op=AND(w2034, w2045, w2046, w2039) -> (w2050:bool)
            n6745 = Unbundle By Name(w2051) -> ("Machine ID"=w2049:string)
            n6746 = call "Email alert.vi"("Email log file path"=w2038, "Send email"=w2050, "Machine ID"=w2049, "Mail server"=w2048, "Alarm message"=w2041, "Recipents"=w2047) -> ()  [unwired: 6 in]
          }
          frame #3 {
            n6747 = local read "Specimen I out of bound"() -> (w2063:bool)
            n6748 = local read "BD1 out of bound"() -> (w2062:bool)
            n6749 = local read "BD2 out of bound"() -> (w2061:bool)
            n6750 = local read "Milling I out of bound"() -> (w2060:bool)
            n6751 = local read "Alert Settings"() -> (w2083:T36)
            n6752 = Select(t="Specimen ", s=w2063, f="") -> (s? t:f=w2070:string)
            n6753 = Select(t="BD1 ", s=w2062, f="") -> (s? t:f=w2068:string)
            n6754 = Select(t="BD2 ", s=w2061, f="") -> (s? t:f=w2067:string)
            n6755 = Select(t="Milling ", s=w2060, f="") -> (s? t:f=w2066:string)
            n6756 = Concatenate Strings("FIB CL ", w2070, w2068, w2067, w2066, "currents out of bound") -> (w2064:string)
            n6757 = local read "FIB"() -> (w2079:bool)
            n6758 = Unbundle By Name(w2083) -> ("FIB CL current alarm"=w2082:bool)
            n6759 = local read "FIB CL I alarm active"() -> (w2084:bool)
            n6760 = local read "Email Alert Recipients"() -> (w2085:string[])
            n6761 = local read "Mail server"() -> (w2086:string)
            n6762 = local read "Hardware Configuration"() -> (w2088:T25)
            n6763 = local read "Email Log Files"() -> (w2080:path)
            n6764 = Unbundle By Name(w2088) -> ("Machine ID"=w2087:string)
            n6765 = Compound Arithmetic op=AND(w2079, w2082, w2084) -> (w2081:bool)
            n6766 = call "Email alert.vi"("Email log file path"=w2080, "Send email"=w2081, "Machine ID"=w2087, "Mail server"=w2086, "Alarm message"=w2064, "Recipents"=w2085) -> ()  [unwired: 6 in]
            n6767 = case shown="True" w2081 {
              frame False {
              }
              frame True {
                n6768 = stacked-sequence {
                  frame #0 {
                    n6769 = Wait (ms)(milliseconds to wait=u32 200) -> ()  [unwired: 1 out]
                  }
                  frame #1 {
                    n6770 = local write "FIB CL I alarm active"(FALSE ("E-mail test")) -> ()
                    n6771 = local write "FIB CL I out of bound counts"(u8 0 ("Specimen I out of bound counts")) -> ()
                  }
                }
              }
            }
          }
          frame #4 {
            n6772 = local read "Alert Settings"() -> (w2096:T36)
            n6773 = local read "FIB"() -> (w2092:bool)
            n6774 = Unbundle By Name(w2096) -> ("Beam Dump 1 alarm"=w2095:bool)
            n6775 = local read "Beam dump at zero"() -> (w2097:bool)
            n6776 = local read "Email Alert Recipients"() -> (w2099:string[])
            n6777 = local read "Mail server"() -> (w2100:string)
            n6778 = local read "Hardware Configuration"() -> (w2102:T25)
            n6779 = local read "Email Log Files"() -> (w2093:path)
            n6780 = Compound Arithmetic op=AND(w2092, w2095, w2097) -> (w2094:bool)
            n6781 = Unbundle By Name(w2102) -> ("Machine ID"=w2101:string)
            n6782 = call "Email alert.vi"("Email log file path"=w2093, "Send email"=w2094, "Machine ID"=w2101, "Mail server"=w2100, "Alarm message"="Beam dump current at or near zero", "Recipents"=w2099) -> ()  [unwired: 6 in]
            n6783 = case shown="True" w2094 {
              frame False {
              }
              frame True {
                n6784 = stacked-sequence {
                  frame #0 {
                    n6785 = Wait (ms)(milliseconds to wait=u32 200) -> ()  [unwired: 1 out]
                  }
                  frame #1 {
                    n6786 = local write "Beam dump at zero"(FALSE ("E-mail test")) -> ()
                  }
                }
              }
            }
          }
          frame #5 {
